vi "Main.vi"() -> ()   [LabVIEW 2014]
uses:
  UI_TimeSelector/UI_TimeSelector.xctl
panel:
  out "Peroid":cluster{"start":timestamp, "end":timestamp} {"start" format="%<%H:%M:%S\n%x>T"; "end" format="%<%H:%M:%S\n%x>T"}
  in  "stop":bool
  out "Time Stamp":timestamp format="%<%H:%M:%S\n%x>T"
  in  "Mode":T1(ring)
  in  "UI_DaySelector":timestamp(xcontrol)
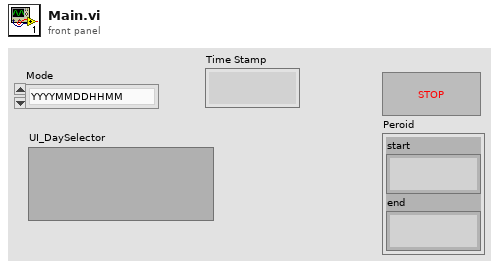
[diagram p1: front panel]
types:
  T1 = enum16{"YYYYMMDDHHMM", "YYYYMMDDHHMMSS", "YYYY", "YYYYMM", "YYYYMMDD", "HHMM", "HHMMSS"}
  T2 = typedef "UI_TimeSelector.xctl/DEF-Mode.ctl" = enum16{"YYYYMMDDHHMM", "YYYYMMDDHHMMSS", "YYYY", "YYYYMM", "YYYYMMDD", "HHMM", "HHMMSS"}
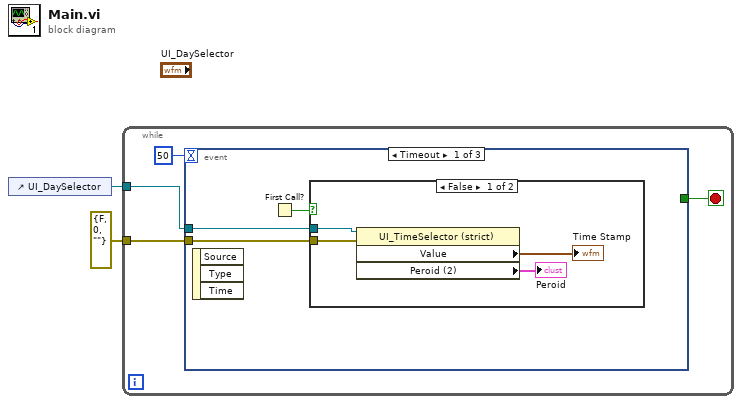
[diagram p0: block diagram]
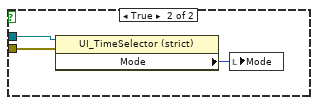
[diagram p2: hidden frame]
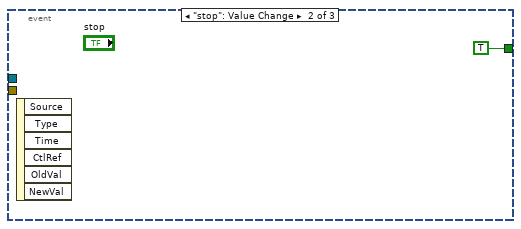
[diagram p3: hidden frame]
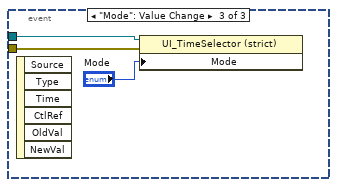
[diagram p4: hidden frame]
diagram:
  n1 = control-ref of="UI_DaySelector"() -> (w2:refnum<vi>)
  n2 = while {
    tunnel: errorcluster {"status"=FALSE, "code"=0, "source"=""} ("error out") -> [w4]
    tunnel: w2 -> [w5]
    stop <- w3 stop-if-true
    n3 = event shown="[0] Timeout" {
      selector: _ -> [_ _ _]
      dyn-events: _ -> [_ _ _]
      timeout: 50 -> [_ _ _]
      tunnel: w5 -> [w9 _ w20]
      tunnel: w4 -> [w8 _ w19]
      tunnel: [_ TRUE _] -> w3
      event Timeout {
        n4 = event-data() -> ()  [unwired: 1 in, 3 out]
        n5 = First Call?() -> (First Call?: T/F=w7:bool)
        n6 = case shown="False" w7 {
          tunnel: w9 -> [w13 w15]
          tunnel: w8 -> [w12 w14]
          frame False {
            n7 = property class="UI_TimeSelector (strict)"(reference=w13, error in=w12) -> ("Value"=→"Time Stamp":timestamp, "Peroid (2)"=→"Peroid":cluster{"start":timestamp, "end":timestamp})  [unwired: 2 out]
          }
          frame True {
            n8 = property class="UI_TimeSelector (strict)"(reference=w15, error in=w14) -> ("Mode"=w16:T2)  [unwired: 2 out]
            n9 = local write "Mode"(w16) -> ()
          }
        }
      }
      event "stop": Value Change {
        n10 = event-data() -> ()  [unwired: 1 in, 6 out]
      }
      event "Mode": Value Change {
        n11 = event-data() -> ()  [unwired: 1 in, 6 out]
        n12 = property on="Property Node" class="UI_TimeSelector (strict)"(reference=w20, error in=w19, "Mode"="Mode") -> ()  [unwired: 2 out]
      }
    }
  }
